vi "Pixy Parser.vi"(0 "Array":u8[](array[numeric])) -> (1 "Array 2":T1(array[cluster]), 2 "Objects Found":u16, 3 "Completed?":bool)   [LabVIEW 2016]
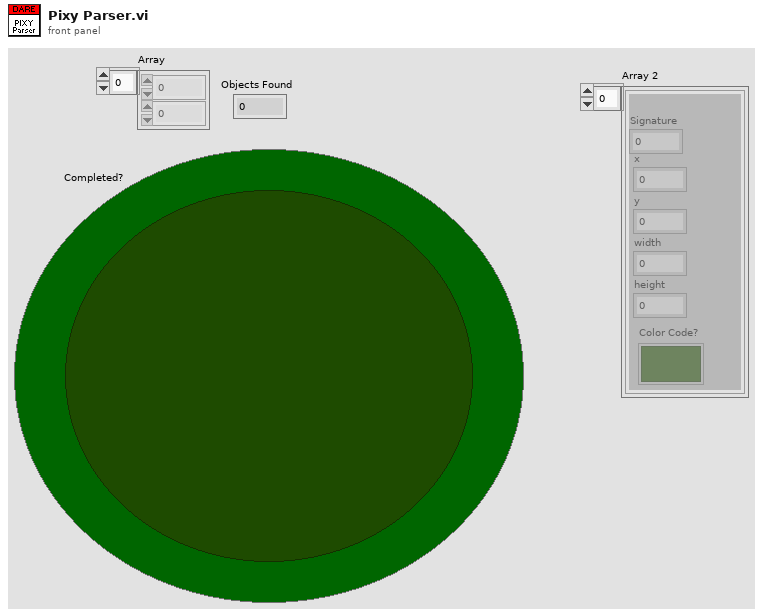
[diagram p1: front panel]
types:
  T1 = cluster{"x":u16, "y":u16, "width":u16, "height":u16, "Signature":u16, "Color Code?":bool}[]
  T2 = cluster{"x":u16, "y":u16, "width":u16, "height":u16, "Signature":u16, "Color Code?":bool}
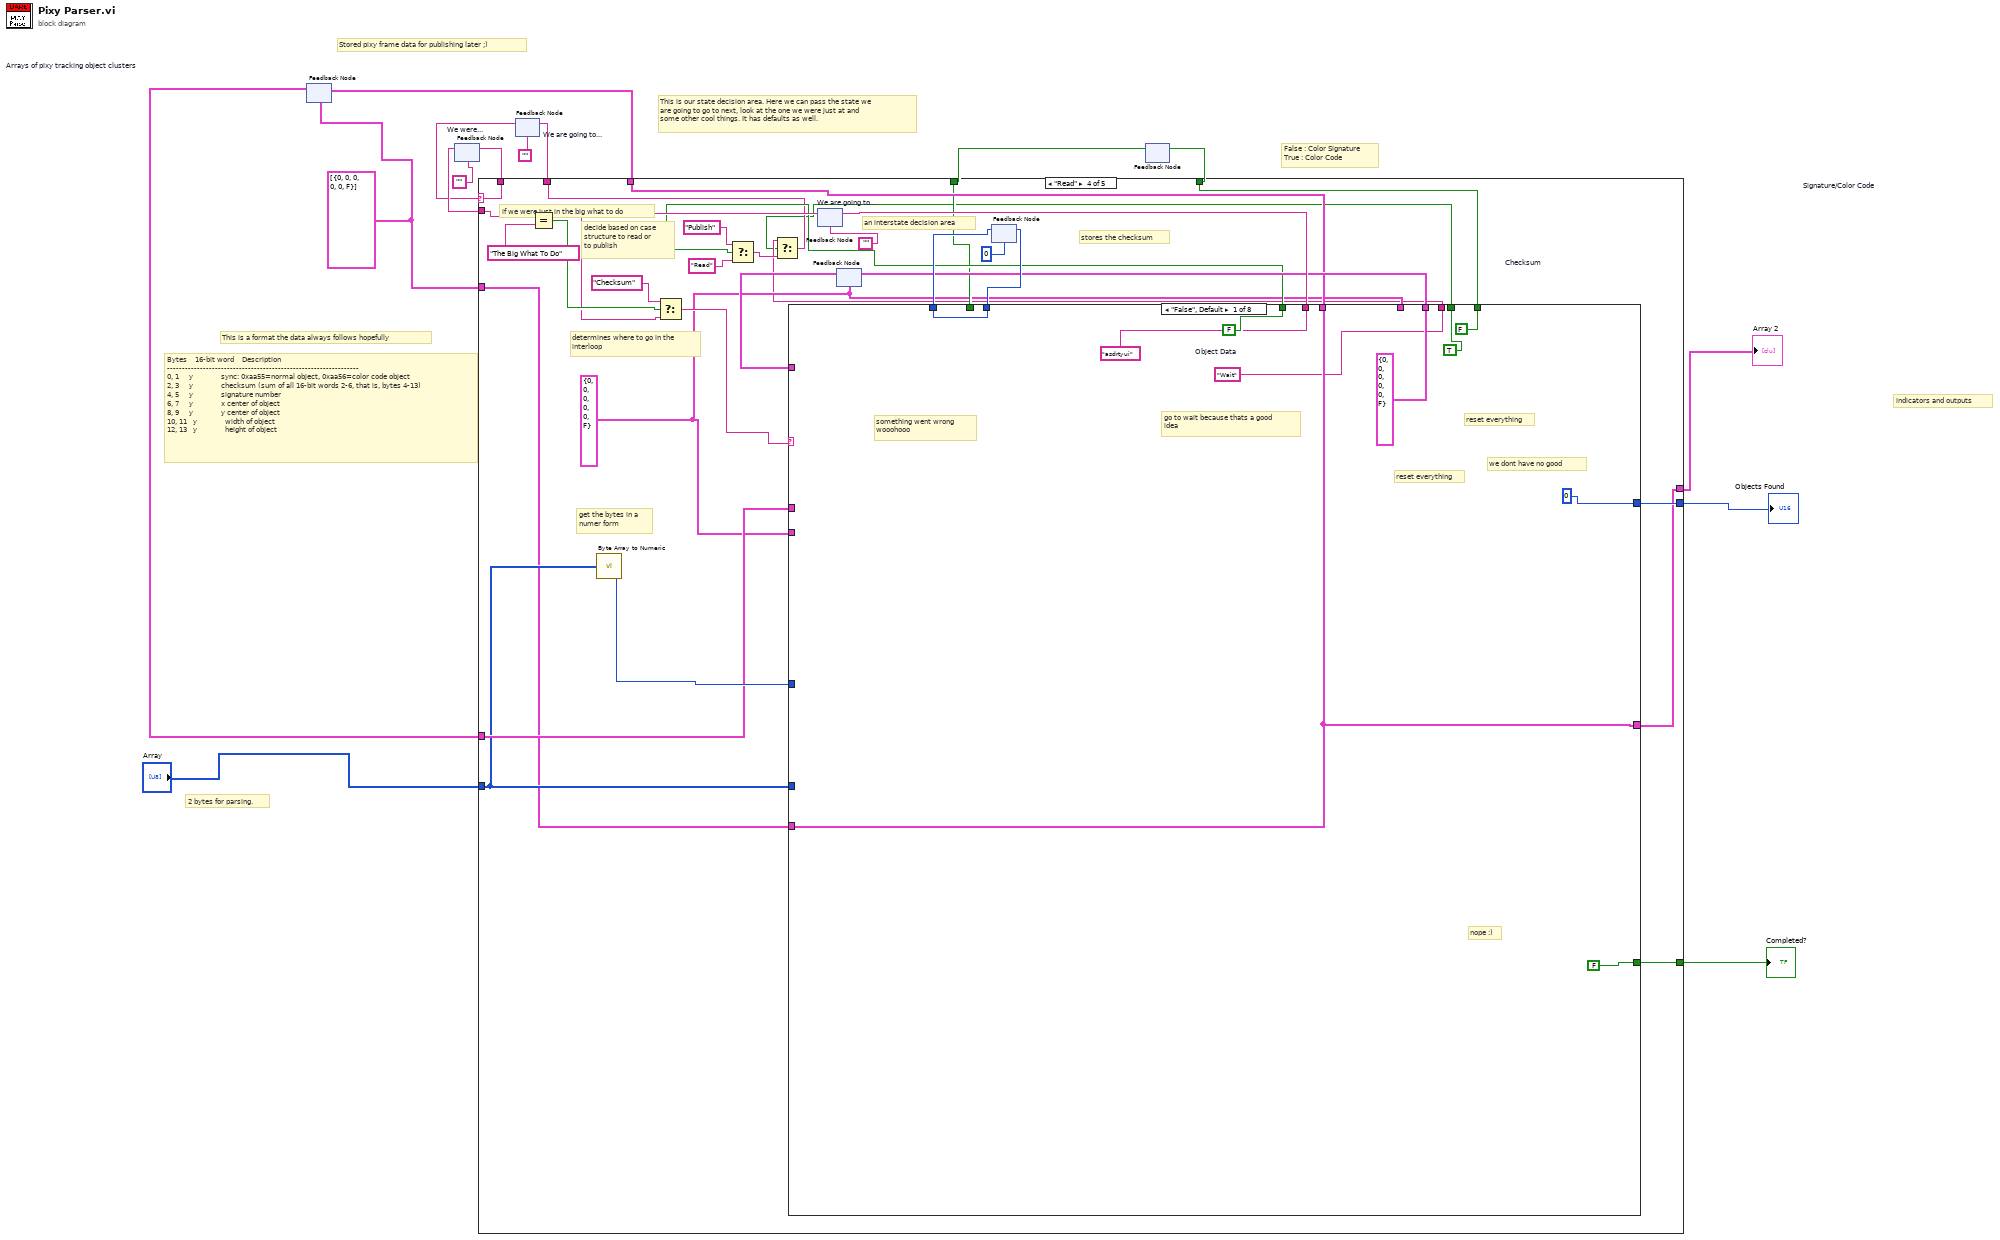
[diagram p0: block diagram]
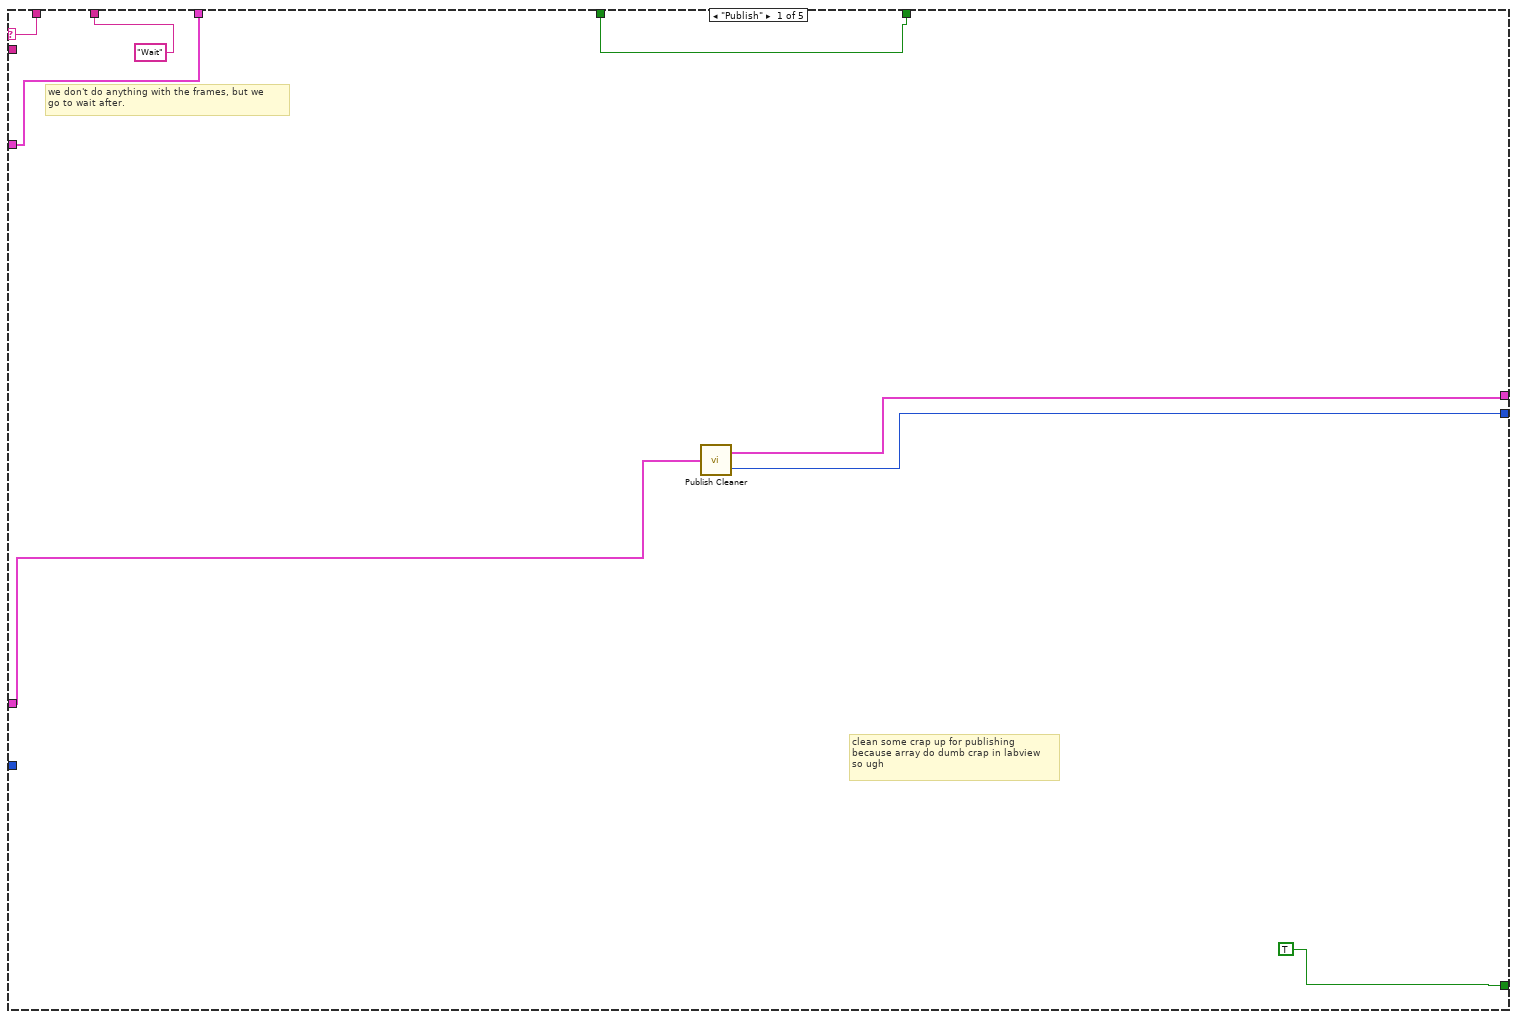
[diagram p2: hidden frame]
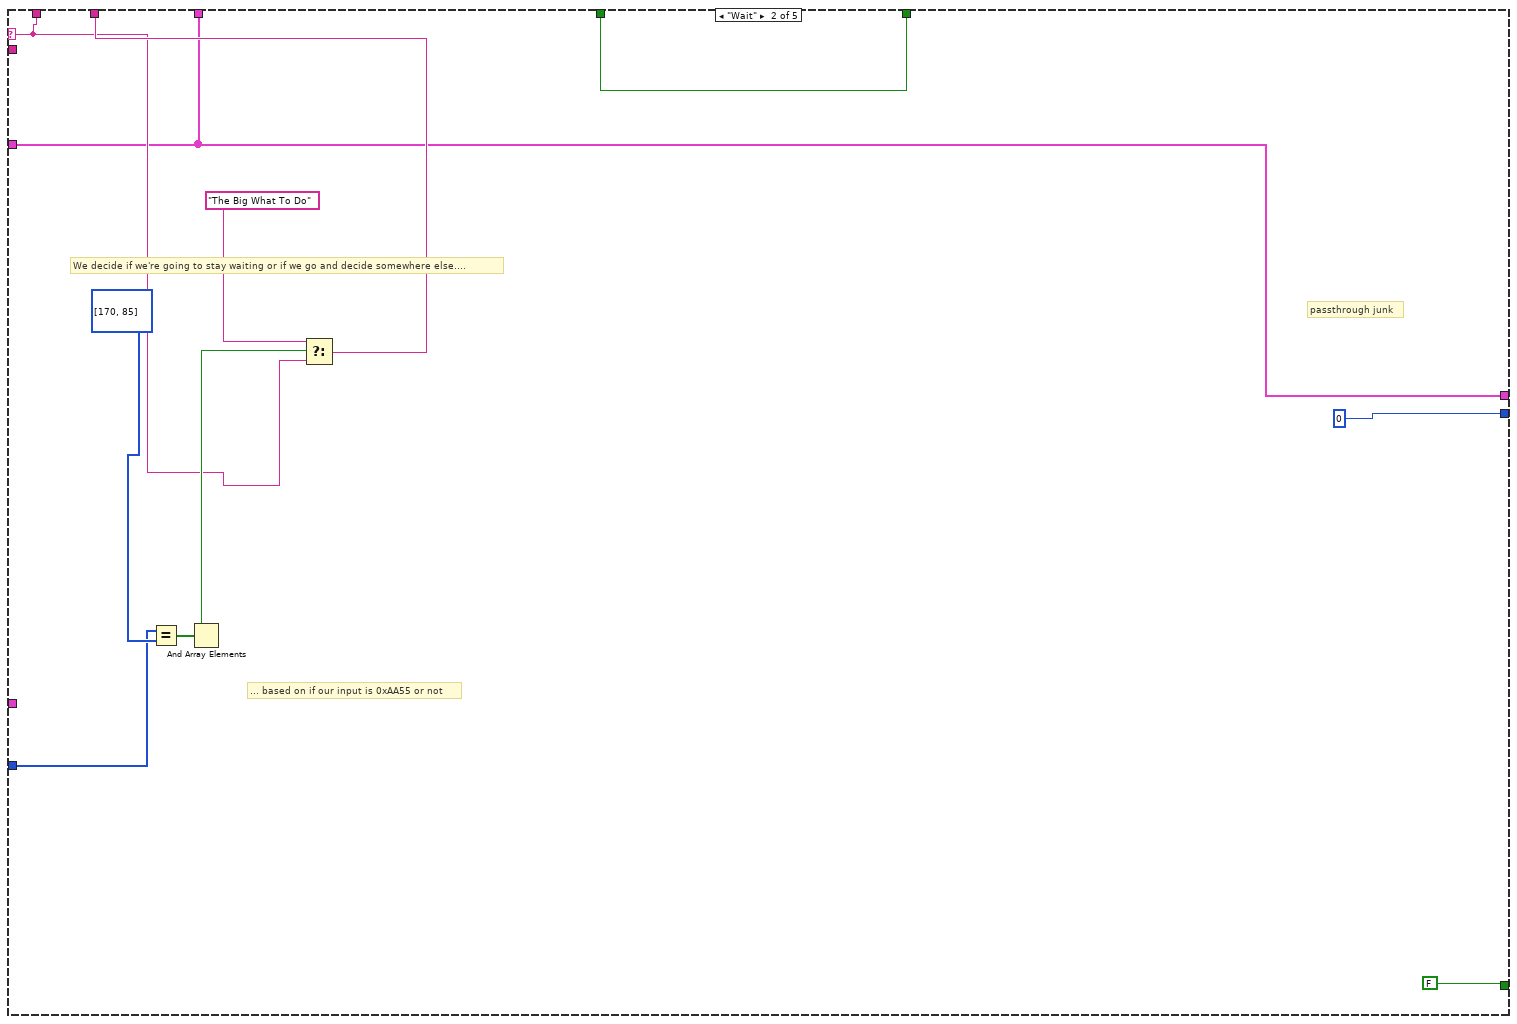
[diagram p3: hidden frame]
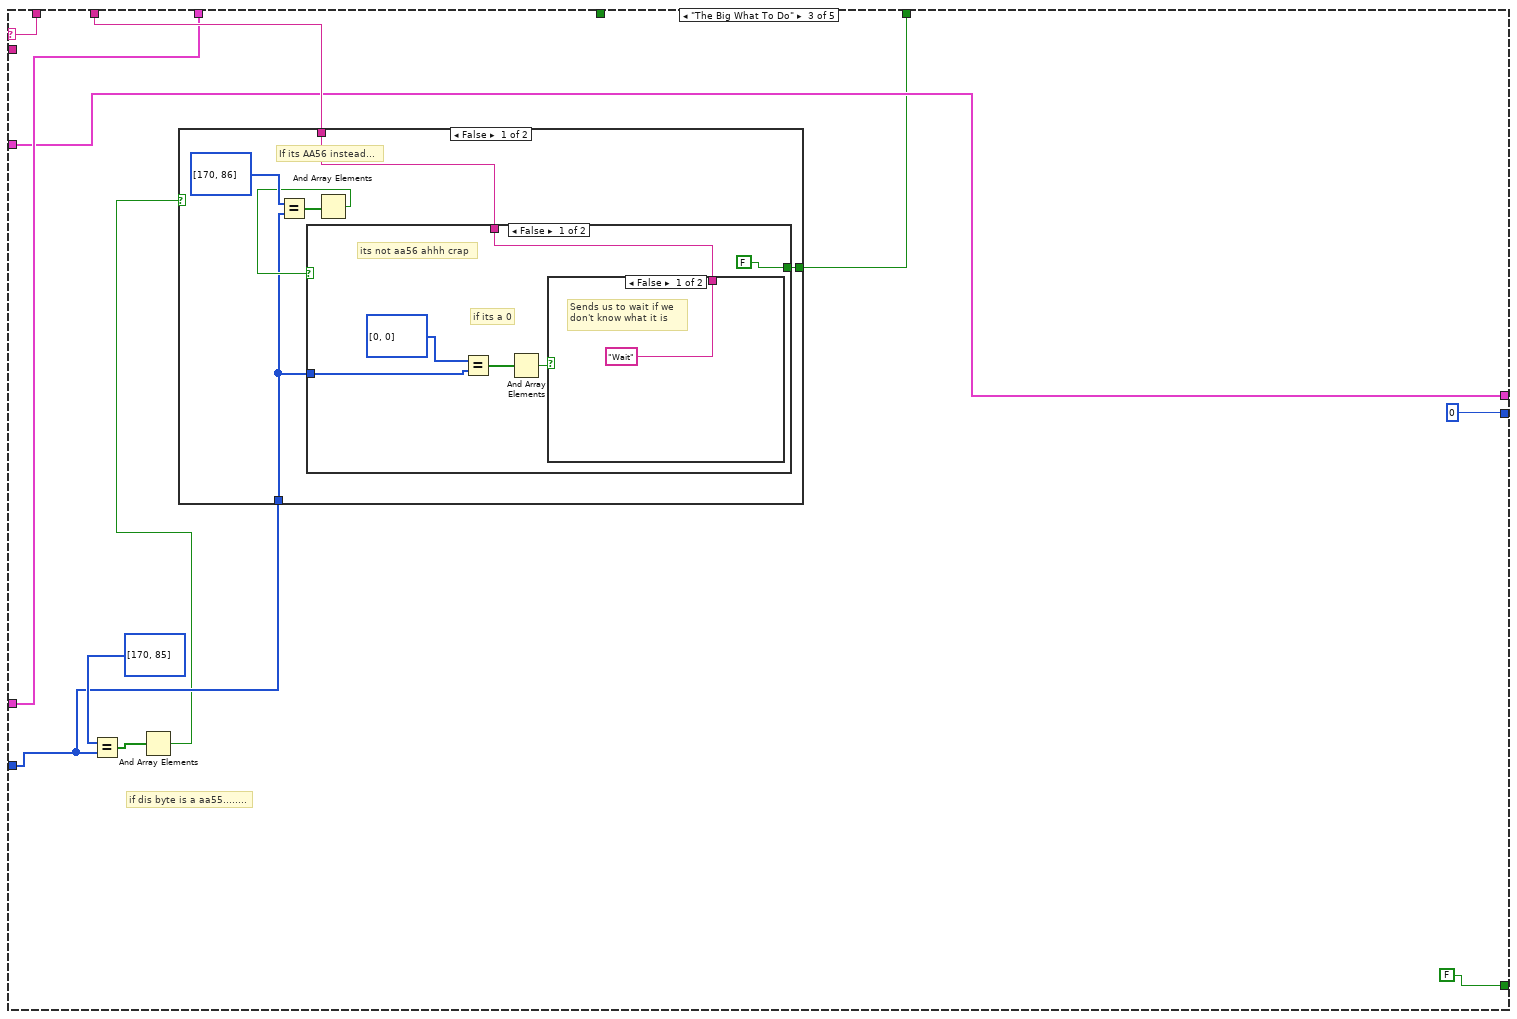
[diagram p4: hidden frame]
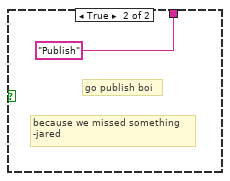
[diagram p5: hidden frame]
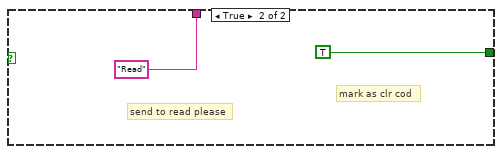
[diagram p6: hidden frame]
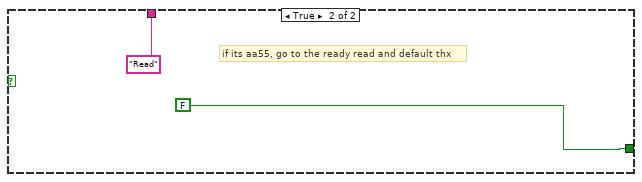
[diagram p7: hidden frame]
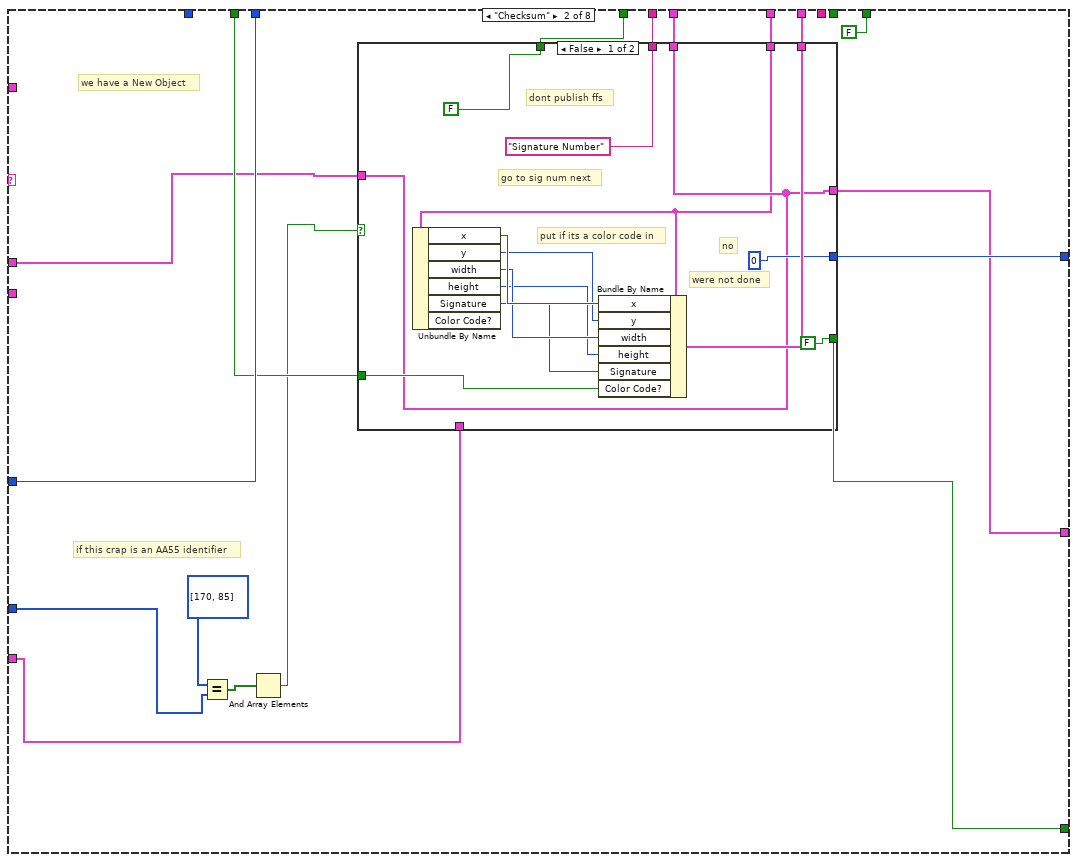
[diagram p8: hidden frame]
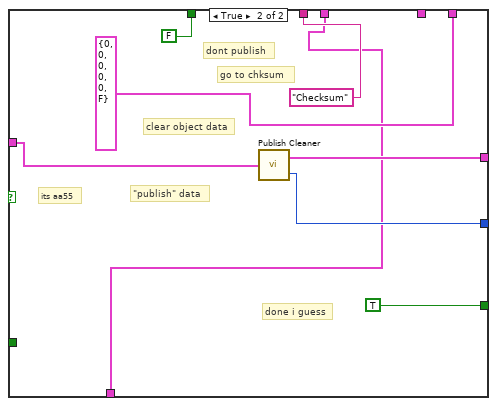
[diagram p9: hidden frame]
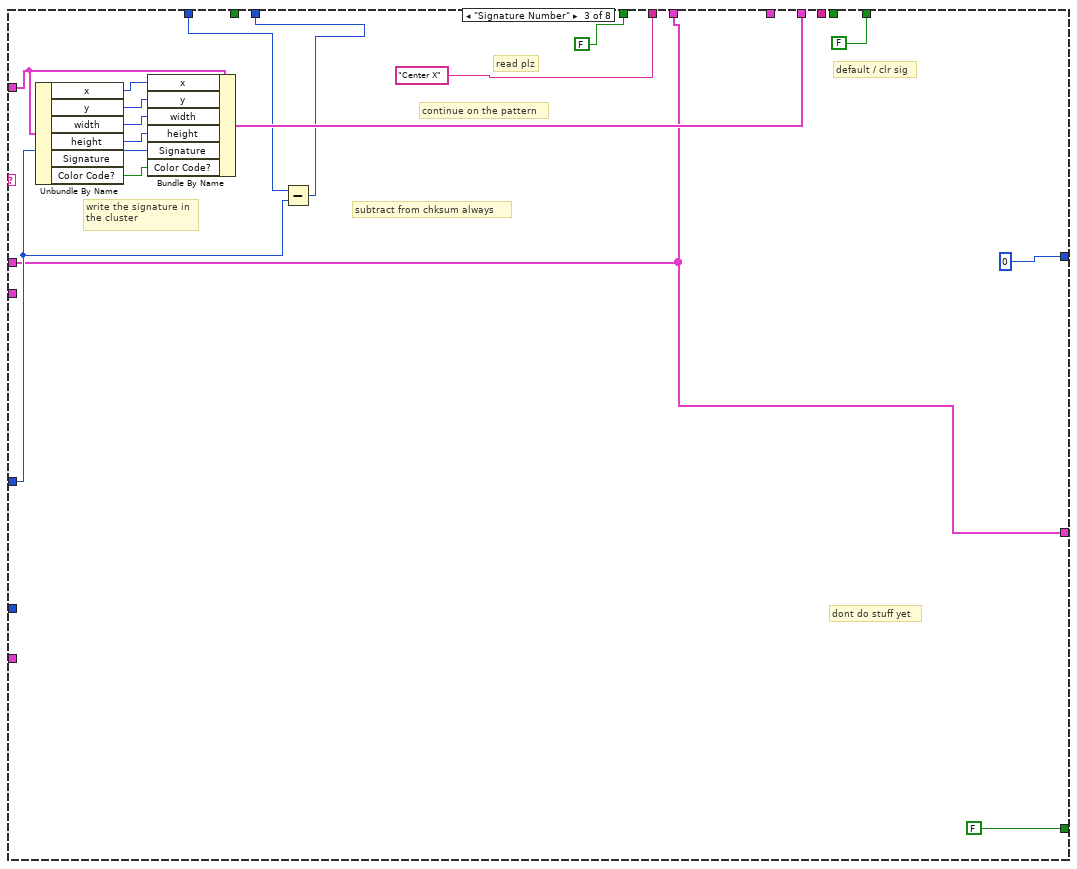
[diagram p10: hidden frame]
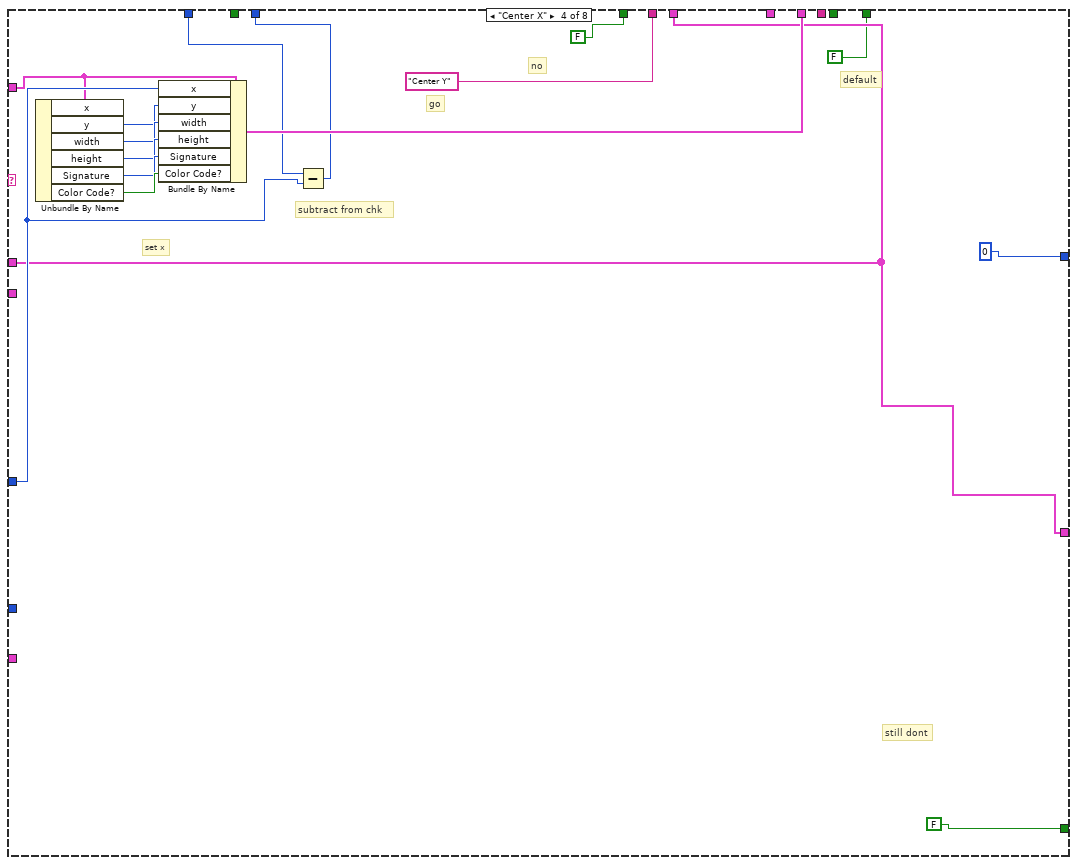
[diagram p11: hidden frame]
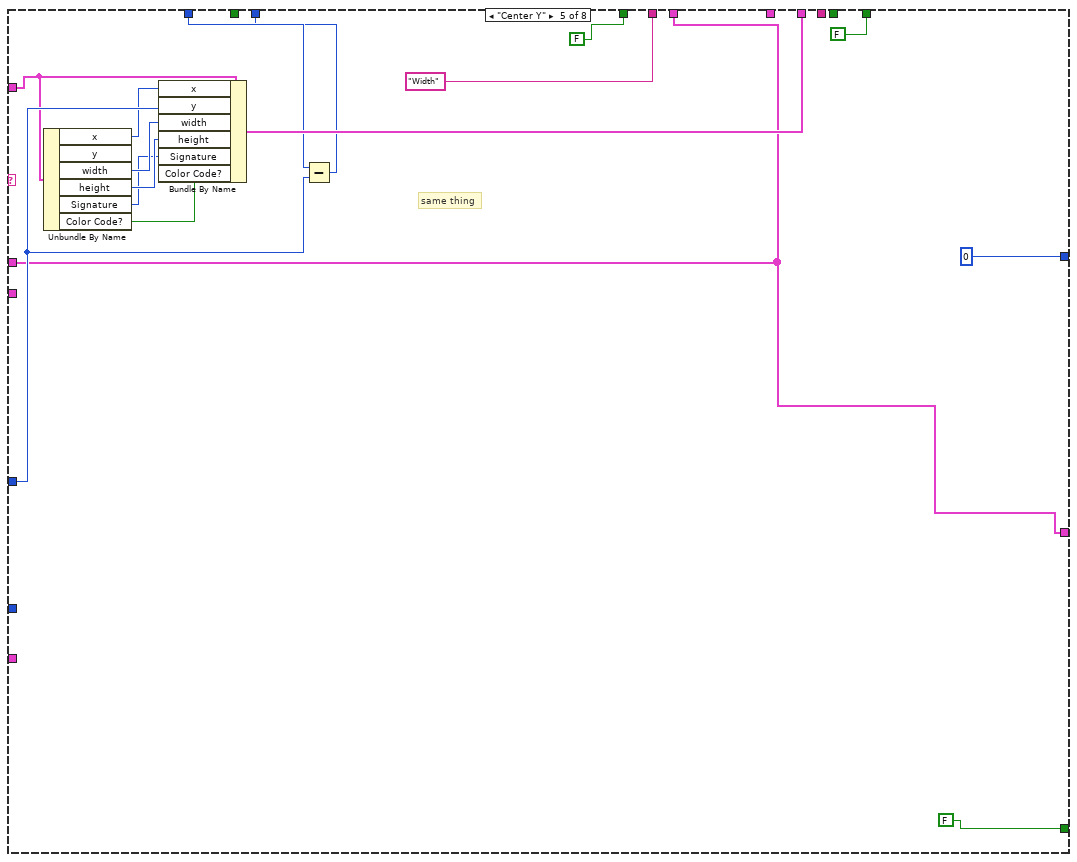
[diagram p12: hidden frame]
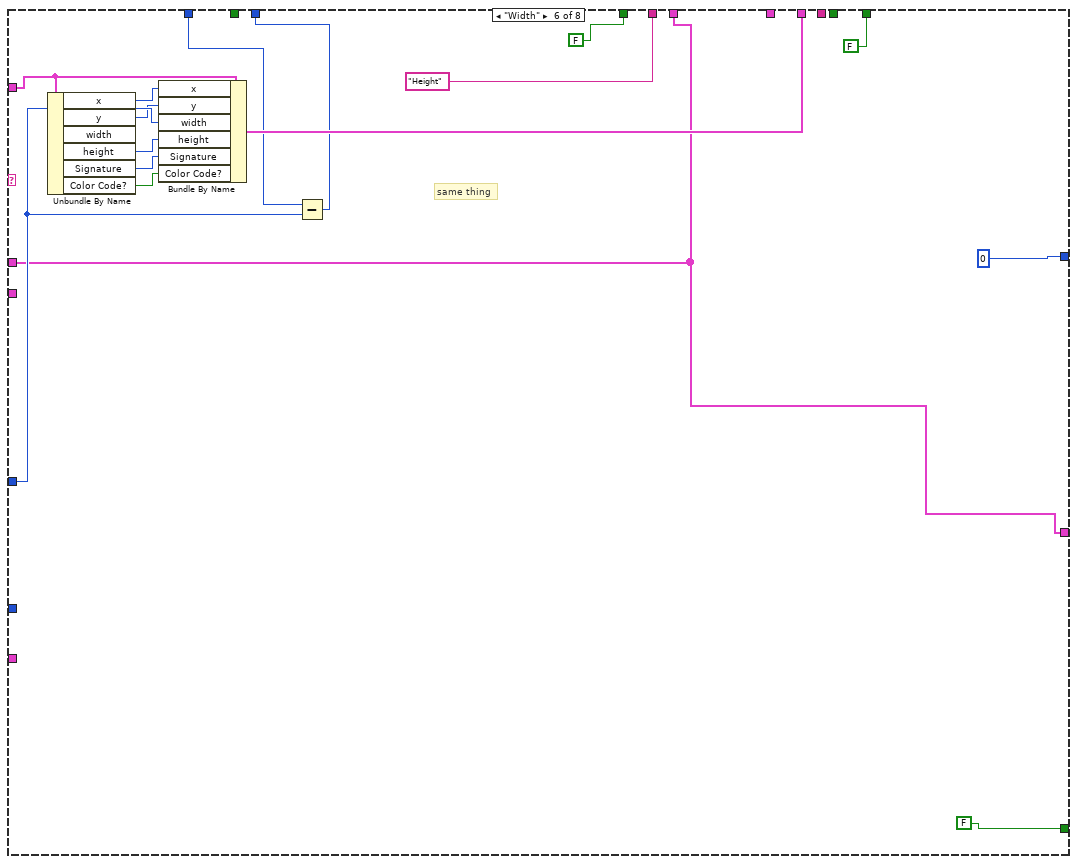
[diagram p13: hidden frame]
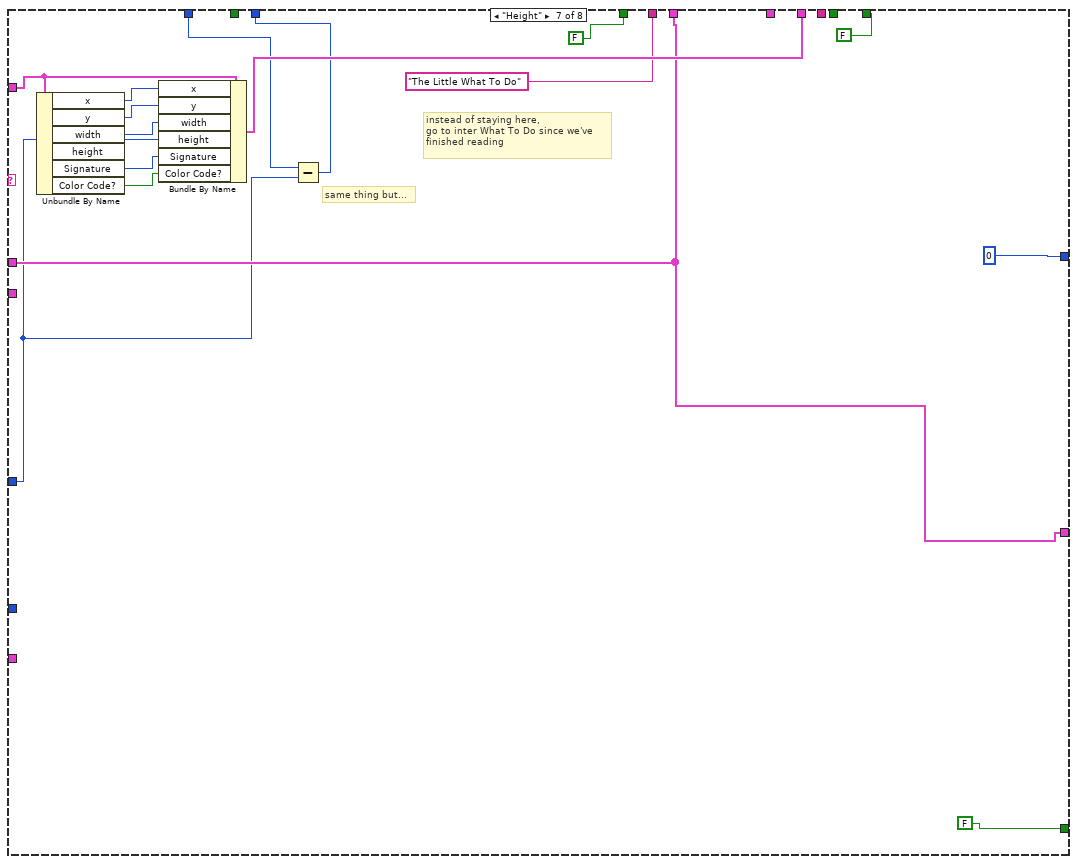
[diagram p14: hidden frame]
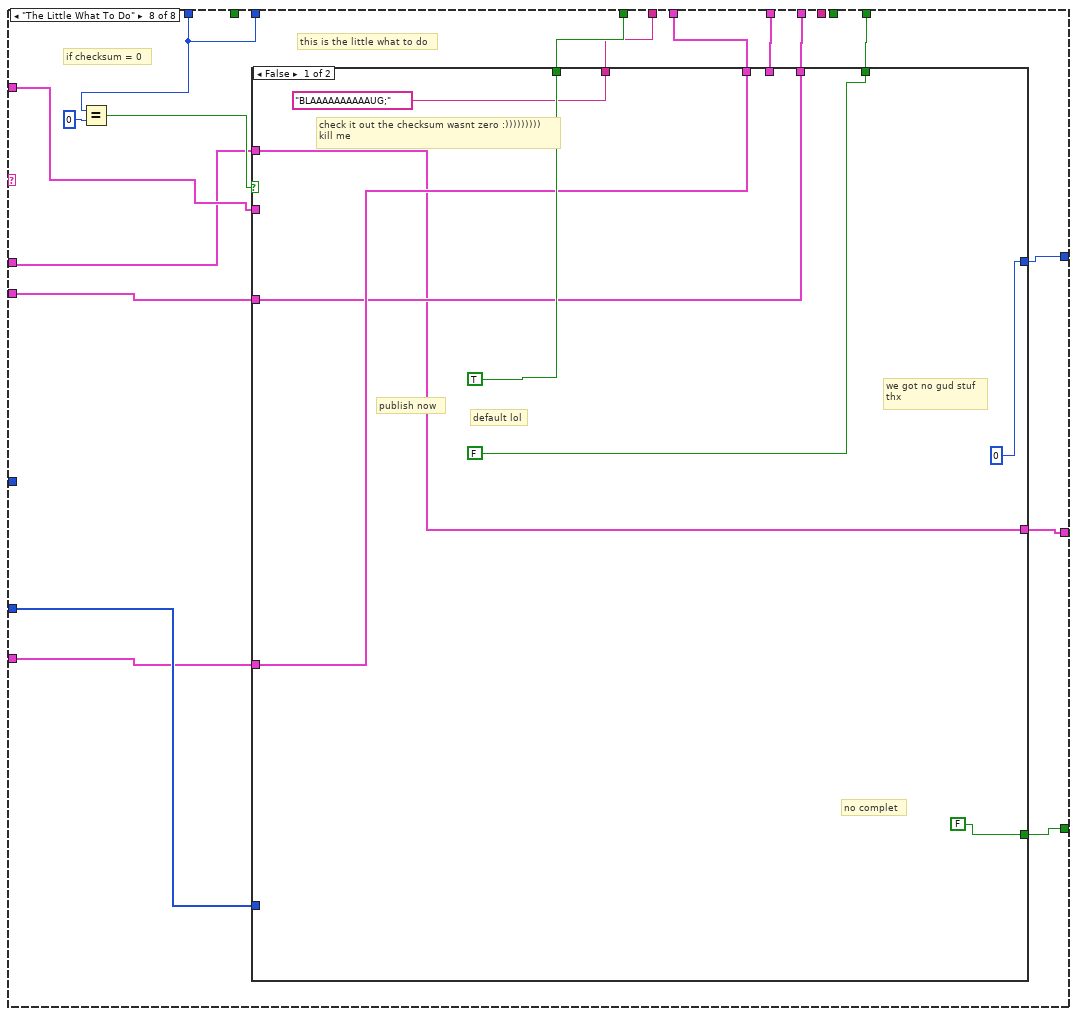
[diagram p15: hidden frame]
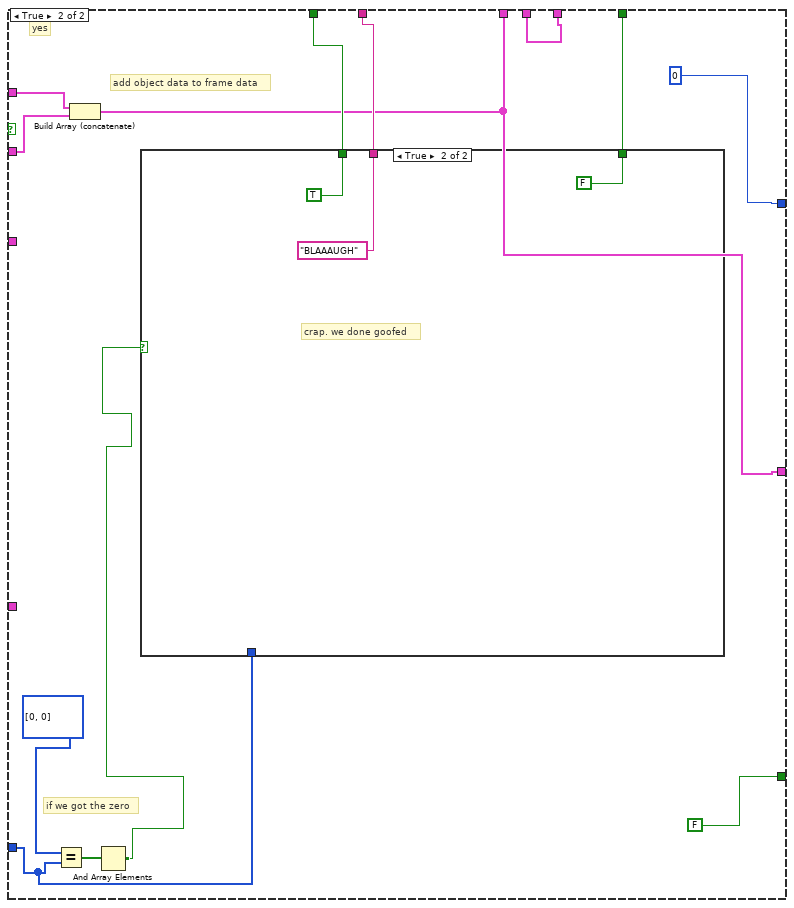
[diagram p16: hidden frame]
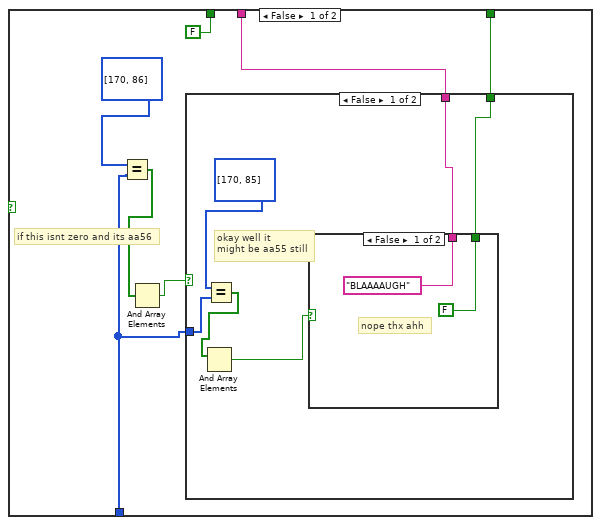
[diagram p17: hidden frame]
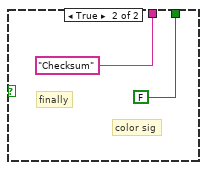
[diagram p18: hidden frame]
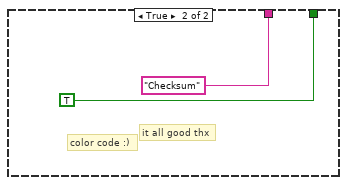
[diagram p19: hidden frame]
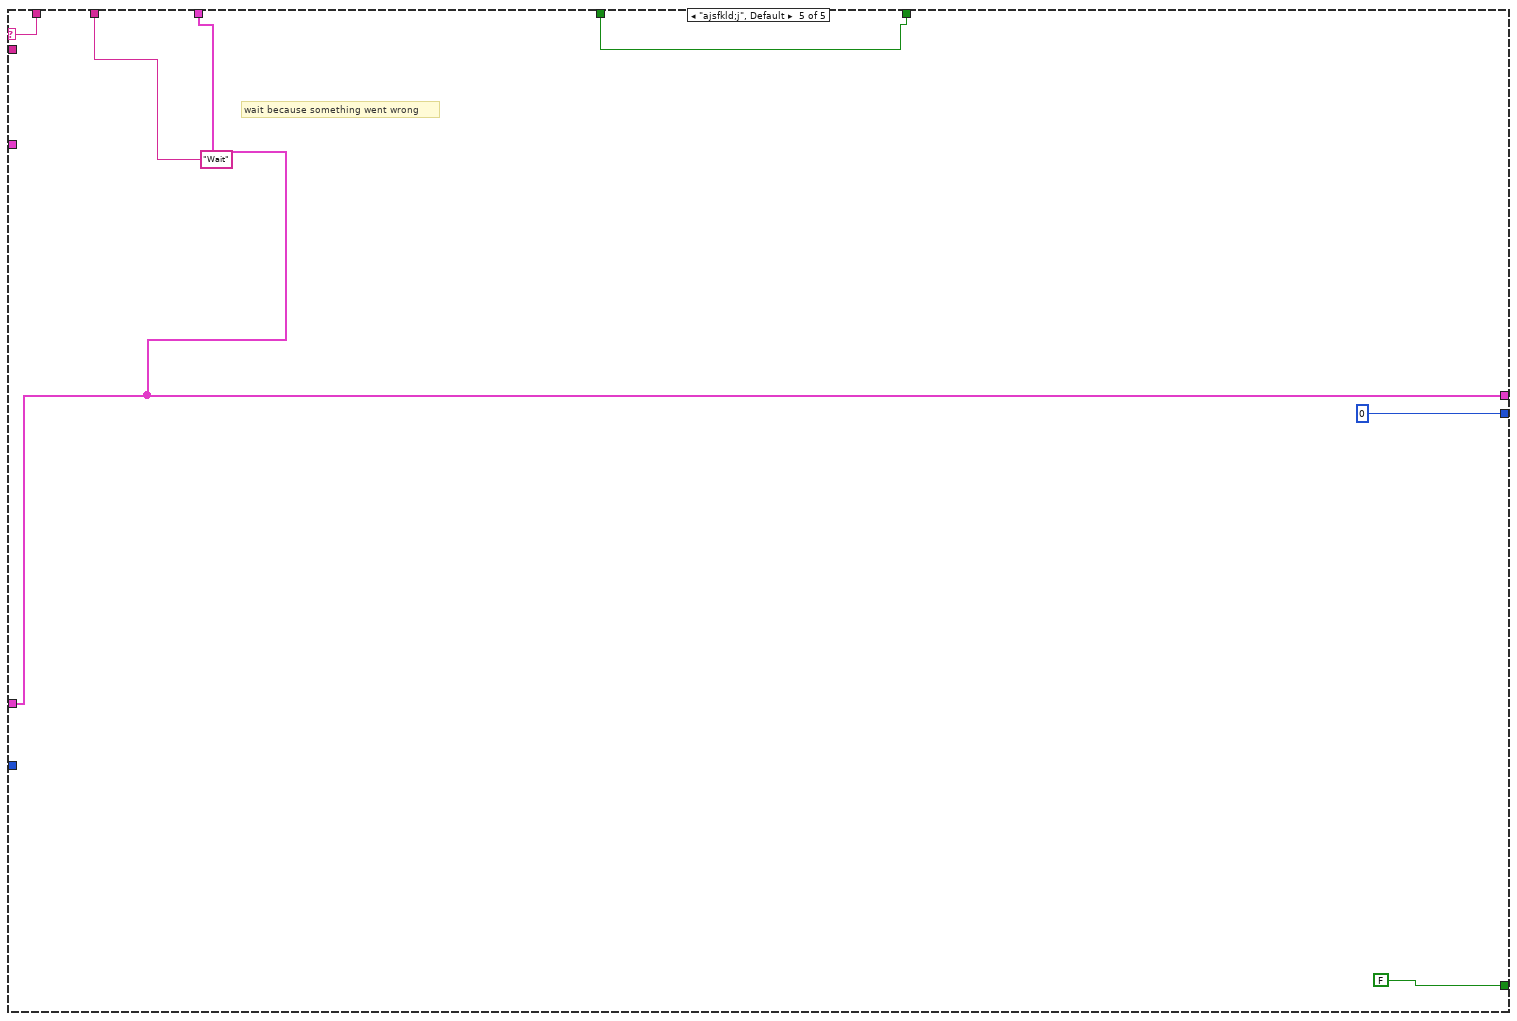
[diagram p20: hidden frame]
diagram:
  w3 = T1 [{"x"=0, "y"=0, "width"=0, "height"=0, "Signature"=0, "Color Code?"=FALSE}] ("Array 3")
  # "indicators and outputs"
  # "This is a format the data always follows hopefully"
  # "Stored pixy frame data for publishing later ;)"
  # "This is our state decision area. Here we can pass the state we\nare going to go to next, look at the one we were just at and\nsome other cool things. It has defaults as well."
  # "2 bytes for parsing."
  # "False : Color Signature\nTrue : Color Code"
  # "Bytes    16-bit word    Description\n----------------------------------------------------------------\n0, 1     y              sync: 0xaa55=normal object, 0xaa56=color code object\n2, 3     y              checksum (sum of all 16-bit words 2-6, that is, bytes 4-13)\n4, 5     y              signature number\n6, 7     y              x center of object\n8, 9     y              y center of object\n10, 11   y              width of object\n12, 13   y              height of object"
  n1 = feedback #1 "Arrays of pixy tracking object clusters"(w3) -> (w15:T1)
  n2 = feedback #2 "We were..."("") -> (w12:string)
  n3 = feedback #3 "We are going to..."("") -> (w10:string)
  n4 = feedback #4 "Signature/Color Code"() -> (w2:bool)  [unwired: 1 in]
  n5 = case shown="\"Read\"" w10 {
    selector: w10 -> [w21 w28 w39 w93 w285]
    tunnel: w15 -> [w23 _ w40 w76 w286]
    tunnel: [w18 w26 w38 w70 w286] -> w4
    tunnel: [TRUE FALSE FALSE w69 FALSE] -> w14
    tunnel: w12 -> [_ _ _ w95 _]
    tunnel: [w21 w28 w39 w93 w285] -> w9
    tunnel: [w19 w26 w40 w78 w286] -> w8
    tunnel: ["Wait" w29 w41 w66 "Wait"] -> w7
    tunnel: "Array" -> [_ w31 w43 w75 _]
    tunnel: [w16 w27 w35 w72 w289] -> w5
    tunnel: w3 -> [w19 w26 w38 w74 _]
    tunnel: w2 -> [w16 w27 _ w73 w289]
    tunnel: [w17 u16 0 u16 0 w71 u16 0] -> w1
    frame "Publish" {
      # "clean some crap up for publishing\nbecause array do dumb crap in labview\nso ugh"
      # "we don't do anything with the frames, but we\ngo to wait after."
      n6 = call "Publish Cleaner.vi"("Array In"=w23) -> ("Cleaned Array"=w18:T1, "Num Objects"=w17:u16)
    }
    frame "Wait" {
      # "passthrough junk"
      # "... based on if our input is 0xAA55 or not"
      # "We decide if we're going to stay waiting or if we go and decide somewhere else...."
      n7 = Equal?(x=w31, y=u8[] [170, 85]) -> (x = y?=w34:bool[])
      n8 = And Array Elements(Boolean array=w34) -> (logical AND=w32:bool)
      n9 = Select(t="The Big What To Do", s=w32, f=w28) -> (s? t:f=w29:string)
    }
    frame "The Big What To Do" {
      # "if dis byte is a aa55........"
      n10 = Equal?(x=u8[] [170, 85], y=w43) -> (x = y?=w45:bool[])
      n11 = And Array Elements(Boolean array=w45) -> (logical AND=w42:bool)
      n12 = case shown="False" w42 {
        tunnel: w43 -> [w47 _]
        tunnel: [w48 "Read"] -> w41
        tunnel: [w46 FALSE] -> w35
        frame False {
          # "If its AA56 instead..."
          n13 = Equal?(x=u8[] [170, 86], y=w47) -> (x = y?=w51:bool[])
          n14 = And Array Elements(Boolean array=w51) -> (logical AND=w49:bool)
          n15 = case shown="False" w49 {
            tunnel: [w53 "Read"] -> w48
            tunnel: w47 -> [w56 _]
            tunnel: [FALSE TRUE] -> w46
            frame False {
              # "if its a 0"
              # "its not aa56 ahhh crap"
              n16 = Equal?(x=u8[] [0, 0], y=w56) -> (x = y?=w55:bool[])
              n17 = And Array Elements(Boolean array=w55) -> (logical AND=w54:bool)
              n18 = case shown="False" w54 {
                tunnel: ["Wait" "Publish"] -> w53
                frame False {
                  # "Sends us to wait if we \ndon't know what it is"
                }
                frame True {
                  # "because we missed something\n-jared"
                  # "go publish boi"
                }
              }
            }
            frame True {
              # "mark as clr cod"
              # "send to read please"
            }
          }
        }
        frame True {
          # "if its aa55, go to the ready read and default thx"
        }
      }
    }
    frame "Read" {
      w68 = T2 {"x"=0, "y"=0, "width"=0, "height"=0, "Signature"=0, "Color Code?"=FALSE} ("Cluster")
      # "if we were just in the big what to do"
      # "determines where to go in the\ninterloop"
      # "decide based on case\nstructure to read or\nto publish"
      # "an interstate decision area"
      # "stores the checksum"
      # "get the bytes in a\nnumer form"
      n19 = Equal?(x=w95, y="The Big What To Do") -> (x = y?=w91:bool)
      n20 = call "Byte Array to Numeric.vi"("2 Bytes"=w75) -> ("U16 Numba"=w85:u16)
      n21 = feedback #5 "We are going to..."("") -> (w89:string)
      n22 = Select(t="Checksum", s=w91, f=w89) -> (s? t:f=w88:string)
      n23 = feedback #6 "Object Data"(w68) -> (w81:T2)
      n24 = feedback #7 "Checksum"(u16 0) -> (w84:u16)
      n25 = case shown="\"False\", Default" w88 {
        tunnel: [w104 w121 w155 w171 w188 w204 w220 w235] -> w86
        tunnel: w85 -> [_ w121 w156 w173 w187 w203 w214 _]
        tunnel: w84 -> [w104 _ w157 w172 w189 w205 w221 w235]
        tunnel: ["asdrtyui" w122 "Center X" "Center Y" "Width" "Height" "The Little What To Do" w236] -> w83
        tunnel: w81 -> [_ _ w149 w165 w181 w197 w212 w234]
        tunnel: [T2 {"x"=0, "y"=0, "width"=0, "height"=0, "Signature"=0, "Color Code?"=FALSE} ("Cluster") w117 w159 w175 w191 w207 w223 w231] -> w80
        tunnel: [w99 w108 w153 w168 w183 w198 w215 w238] -> w78
        tunnel: [FALSE w120 FALSE FALSE FALSE FALSE FALSE w237] -> w77
        tunnel: w76 -> [_ w112 w153 w168 w183 w198 w215 w233]
        tunnel: w75 -> [_ w115 _ _ _ _ _ w232]
        tunnel: w68 -> [_ w119 _ _ _ _ _ w230]
        tunnel: w74 -> [w99 w107 _ _ _ _ _ w229]
        tunnel: w73 -> [_ w118 _ _ _ _ _ _]
        tunnel: [FALSE FALSE FALSE FALSE FALSE FALSE FALSE w228] -> w72
        tunnel: [u16 0 w111 u16 0 u16 0 u16 0 u16 0 u16 0 w224] -> w71
        tunnel: [w99 w110 w153 w168 w183 w198 w215 w226] -> w70
        tunnel: [FALSE w109 FALSE FALSE FALSE FALSE FALSE w225] -> w69
        tunnel: w68 -> [_ _ _ _ _ _ _ w227]
        tunnel: ["Wait" _ _ _ _ _ _ _] -> w65
        tunnel: [TRUE _ _ _ _ _ _ _] -> w64
        frame "False", Default {
          # "nope :)"
          # "we dont have no good"
          # "reset everything"
          # "reset everything"
          # "go to wait because thats a good\nidea"
          # "something went wrong\nwooohooo"
        }
        frame "Checksum" {
          # "if this crap is an AA55 identifier"
          # "we have a New Object"
          n26 = Equal?(x=u8[] [170, 85], y=w115) -> (x = y?=w114:bool[])
          n27 = And Array Elements(Boolean array=w114) -> (logical AND=w113:bool)
          n28 = case shown="False" w113 {
            tunnel: ["Signature Number" "Checksum"] -> w122
            tunnel: [FALSE FALSE] -> w120
            tunnel: w119 -> [w128 _]
            tunnel: w118 -> [w133 _]
            tunnel: [w132 T2 {"x"=0, "y"=0, "width"=0, "height"=0, "Signature"=0, "Color Code?"=FALSE} ("Cluster")] -> w117
            tunnel: w112 -> [w129 w141]
            tunnel: [u16 0 w143] -> w111
            tunnel: [w129 w142] -> w110
            tunnel: [FALSE TRUE] -> w109
            tunnel: [w129 w136] -> w108
            tunnel: w107 -> [_ w136]
            frame False {
              # "no"
              # "were not done"
              # "put if its a color code in"
              # "go to sig num next"
              # "dont publish ffs"
              n29 = Unbundle By Name(w128) -> ("x"=w127:u16, "y"=w126:u16, "width"=w125:u16, "height"=w124:u16, "Signature"=w123:u16)  [unwired: 1 out]
              n30 = Bundle By Name(cluster=w128, "x"=w127, "y"=w126, "width"=w125, "height"=w124, "Signature"=w123, "Color Code?"=w133) -> (w132:T2)
            }
            frame True {
              # "done i guess"
              # "\"publish\" data"
              # "dont publish"
              # "go to chksum"
              # "clear object data"
              # "its aa55"
              n31 = call "Publish Cleaner.vi"("Array In"=w141) -> ("Cleaned Array"=w142:T1, "Num Objects"=w143:u16)
            }
          }
        }
        frame "Signature Number" {
          # "dont do stuff yet"
          # "default / clr sig"
          # "read plz"
          # "continue on the pattern"
          # "subtract from chksum always"
          # "write the signature in\nthe cluster"
          n32 = Unbundle By Name(w149) -> ("x"=w148:u16, "y"=w147:u16, "width"=w146:u16, "height"=w145:u16, "Color Code?"=w144:bool)  [unwired: 1 out]
          n33 = Bundle By Name(cluster=w149, "x"=w148, "y"=w147, "width"=w146, "height"=w145, "Signature"=w156, "Color Code?"=w144) -> (w159:T2)
          n34 = Subtract(x=w157, y=w156) -> (x-y=w155:u16)
        }
        frame "Center X" {
          # "default"
          # "no"
          # "go"
          # "subtract from chk"
          # "set x"
          # "still dont"
          n35 = Unbundle By Name(w165) -> ("y"=w160:u16, "width"=w161:u16, "height"=w162:u16, "Signature"=w163:u16, "Color Code?"=w164:bool)  [unwired: 1 out]
          n36 = Bundle By Name(cluster=w165, "x"=w173, "y"=w160, "width"=w161, "height"=w162, "Signature"=w163, "Color Code?"=w164) -> (w175:T2)
          n37 = Subtract(x=w172, y=w173) -> (x-y=w171:u16)
        }
        frame "Center Y" {
          # "same thing"
          n38 = Unbundle By Name(w181) -> ("x"=w180:u16, "width"=w179:u16, "height"=w178:u16, "Signature"=w177:u16, "Color Code?"=w176:bool)  [unwired: 1 out]
          n39 = Bundle By Name(cluster=w181, "x"=w180, "y"=w187, "width"=w179, "height"=w178, "Signature"=w177, "Color Code?"=w176) -> (w191:T2)
          n40 = Subtract(x=w189, y=w187) -> (x-y=w188:u16)
        }
        frame "Width" {
          # "same thing"
          n41 = Unbundle By Name(w197) -> ("x"=w196:u16, "y"=w195:u16, "height"=w194:u16, "Signature"=w193:u16, "Color Code?"=w192:bool)  [unwired: 1 out]
          n42 = Bundle By Name(cluster=w197, "x"=w196, "y"=w195, "width"=w203, "height"=w194, "Signature"=w193, "Color Code?"=w192) -> (w207:T2)
          n43 = Subtract(x=w205, y=w203) -> (x-y=w204:u16)
        }
        frame "Height" {
          # "instead of staying here,\ngo to inter What To Do since we've\nfinished reading"
          # "same thing but..."
          n44 = Unbundle By Name(w212) -> ("x"=w213:u16, "y"=w211:u16, "width"=w210:u16, "Signature"=w209:u16, "Color Code?"=w208:bool)  [unwired: 1 out]
          n45 = Bundle By Name(cluster=w212, "x"=w213, "y"=w211, "width"=w210, "height"=w214, "Signature"=w209, "Color Code?"=w208) -> (w223:T2)
          n46 = Subtract(x=w221, y=w214) -> (x-y=w220:u16)
        }
        frame "The Little What To Do" {
          # "if checksum = 0"
          # "this is the little what to do"
          n47 = Equal?(x=w235, y=u16 0) -> (x = y?=w239:bool)
          n48 = case shown="False" w239 {
            tunnel: [w246 w252] -> w238
            tunnel: [TRUE w257] -> w237
            tunnel: ["BLAAAAAAAAAAUG;" w255] -> w236
            tunnel: w234 -> [_ w261]
            tunnel: w233 -> [w243 w260]
            tunnel: w232 -> [_ w256]
            tunnel: [w244 w254] -> w231
            tunnel: w230 -> [_ w254]
            tunnel: w229 -> [w246 _]
            tunnel: [FALSE w253] -> w228
            tunnel: w227 -> [w244 _]
            tunnel: [w243 w252] -> w226
            tunnel: [u16 0 u16 0] -> w224
            tunnel: [FALSE FALSE] -> w225
            frame False {
              # "no complet"
              # "we got no gud stuf\nthx"
              # "default lol"
              # "publish now"
              # "check it out the checksum wasnt zero :)))))))))\nkill me"
            }
            frame True {
              # "if we got the zero"
              # "add object data to frame data"
              # "yes"
              n49 = Equal?(x=u8[] [0, 0], y=w256) -> (x = y?=w258:bool[])
              n50 = Build Array (concatenate)(w260, w261) -> (w252:T1)
              n51 = And Array Elements(Boolean array=w258) -> (logical AND=w249:bool)
              n52 = case shown="True" w249 {
                tunnel: [FALSE TRUE] -> w257
                tunnel: w256 -> [w263 _]
                tunnel: [w264 "BLAAAUGH"] -> w255
                tunnel: [w262 FALSE] -> w253
                frame False {
                  # "if this isnt zero and its aa56"
                  n53 = Equal?(x=u8[] [170, 86], y=w263) -> (x = y?=w267:bool[])
                  n54 = And Array Elements(Boolean array=w267) -> (logical AND=w266:bool)
                  n55 = case shown="False" w266 {
                    tunnel: [w270 "Checksum"] -> w264
                    tunnel: w263 -> [w273 _]
                    tunnel: [w269 TRUE] -> w262
                    frame False {
                      # "okay well it \nmight be aa55 still"
                      n56 = Equal?(x=u8[] [170, 85], y=w273) -> (x = y?=w272:bool[])
                      n57 = And Array Elements(Boolean array=w272) -> (logical AND=w271:bool)
                      n58 = case shown="False" w271 {
                        tunnel: ["BLAAAAUGH" "Checksum"] -> w270
                        tunnel: [FALSE FALSE] -> w269
                        frame False {
                          # "nope thx ahh"
                        }
                        frame True {
                          # "color sig"
                          # "finally"
                        }
                      }
                    }
                    frame True {
                      # "color code :)"
                      # "it all good thx"
                    }
                  }
                }
                frame True {
                  # "crap. we done goofed"
                }
              }
            }
          }
        }
      }
      n59 = Select(t="Publish", s=w77, f="Read") -> (s? t:f=w67:string)
      n60 = Select(t=w65, s=w64, f=w67) -> (s? t:f=w66:string)
      n61 = feedback-in #5(w83) -> ()
      n62 = feedback-in #6(w80) -> ()
      n63 = feedback-in #7(w86) -> ()
    }
    frame "ajsfkld;j", Default {
      # "wait because something went wrong"
    }
  }
  "Objects Found" <- w1
  "Array 2" <- w4
  "Completed?" <- w14
  n64 = feedback-in #1(w8) -> ()
  n65 = feedback-in #2(w9) -> ()
  n66 = feedback-in #3(w7) -> ()
  n67 = feedback-in #4(w5) -> ()
